vi "Engine - Copy & Script PPLTemplates.vi"(7 "CD Name":string, 8 "error in (no error)":errorcluster, 9 "RT Driver VI Path":path, 10 "RT Driver Folder Path":path, 11 "CD Source Folder Path":path) -> (0 "error out":errorcluster)   [LabVIEW 2020, in "NIVS_Consolidated_CDW_MetaDataObj.lvclass"]
doc: "Via scripting, replace the tempate RTStateVariables control with the new type def across the async and RT driver VIs, and script the compiled settings property into the constants global"
uses:
  NIVS_Consolidated_CDW_MetaDataObj.lvclass
  Common.ctl
  CD Shared lvlib.ctl
  CD Engine lvlib.ctl
  Common.vi
  CD Shared lvlib.vi
  CD Engine lvlib.vi
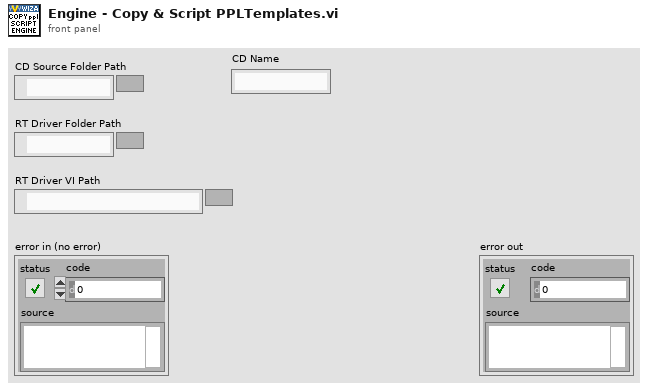
[diagram p1: front panel]
types:
  T1 = typedef "NIVS_Consolidated_CDW_MetaDataObj.lvclass/CD Engine lvlib.ctl" = enum16{"LibraryFileName", "LibraryFolderName", "Engine.FolderName", "Engine.Init.FolderName", "Engine.Run.FolderName", "Engine.Shutdown.FolderName", "Types.FolderName", "Engine.RT Driver VI.TemplatePath", "Engine.RT Driver VI.FileName", "Engine.PPL.RT Driver VI_InlineAsync.FileName", "Engine.RTStateVariables.Name", "Engine.PPL.RTStateVariables.Name", "Engine.RTStateVariables.Name.NoExtension", "Engine.Async.NameExtension", "Engine.Async.TemplateName", "Engine.PPL.Async.TemplateName", "Engine.PPL.Async.InitVSGlobals.Name", "Engine.PPL.RT Driver VI_Inline.FileName"}
  T2 = typedef "NIVS_Consolidated_CDW_MetaDataObj.lvclass/CD Shared lvlib.ctl" = enum16{"LibraryFileName", "LibraryFolderName", "ConstantsVI.VIPathAndName", "Shared.FolderName", "Shared.Types.FolderName", "Shared.Constants.VIName", "Shared.Constants.VITemplateName", "Shared.Constants.VITemplatePathAndName", "Shared.CompiledSettings.RelativePath", "Shared.Constants.RelativePath", "Shared.CompiledSettings.Name", "Shared.CompiledSettings.Name.NoExtension", "Shared.CompiledSettings.ClusterName"}
  T3 = typedef "NIVS_Consolidated_CDW_MetaDataObj.lvclass/Common.ctl" = enum16{"ProjectName", "TemplatesFolderName", "PPLTemplatesFolderName", "ProjectTemplatePathAndName", "ProjectPPLTemplatePathAndName", "TimingAndSyncFolderName", "CustomDeviceFolderName", "PathToTemplates", "PathToPPLTemplates", "PathToExplorerPPLTemplates", "PathToEnginePPLTemplates", "PathToConfigurationFile", "ProjectConfigurationName"}
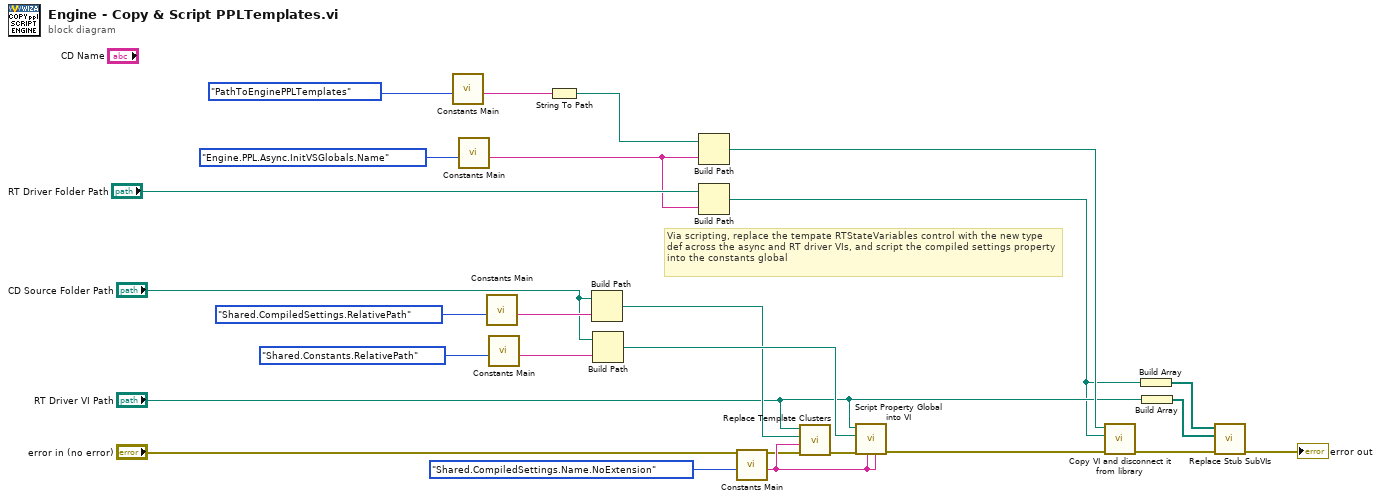
[diagram p0: block diagram]
diagram:
  # "Via scripting, replace the tempate RTStateVariables control with the new type def across the async and RT driver VIs, and script the compiled settings property into the constants global"
  n1 = call-poly "Constants Main.vi"("Action"=Common."PathToEnginePPLTemplates") -> ("Output"=w22:string)  [unwired: 10 in]
  n2 = call-poly "Constants Main.vi"("Action"=CD_Engine_lvlib."Engine.PPL.Async.InitVSGlobals.Name") -> ("Output"=w8:string)  [unwired: 10 in]
  n3 = call-poly "Constants Main.vi"("Action"=CD_Shared_lvlib."Shared.CompiledSettings.RelativePath") -> ("Output"=w19:string)  [unwired: 10 in]
  n4 = call-poly "Constants Main.vi"("Action"=CD_Shared_lvlib."Shared.Constants.RelativePath") -> ("Output"=w17:string)  [unwired: 10 in]
  n5 = String To Path(string=w22) -> (path=w11:path)
  n6 = Build Path(base path="CD Source Folder Path", name or relative path=w19) -> (appended path=w24:path)
  n7 = Build Path(base path="CD Source Folder Path", name or relative path=w17) -> (appended path=w25:path)
  n8 = Build Path(base path=w11, name or relative path=w8) -> (appended path=w10:path)
  n9 = Build Path(base path="RT Driver Folder Path", name or relative path=w8) -> (appended path=w2:path)
  n10 = call-poly "Constants Main.vi"("Action"=CD_Shared_lvlib."Shared.CompiledSettings.Name.NoExtension") -> ("Output"=w14:string)  [unwired: 10 in]
  n11 = call "Replace Template Clusters.vi"("error in (no error)"="error in (no error)", "Control Name"=w14, "Path to Cluster to Replace"=w24, "Path to VI"="RT Driver VI Path") -> ("error out"=w23:errorcluster)  [unwired: 7 in]
  n12 = call "Script Property Global into VI.vi"("GlobalControlName"=w14, "StringConstantToReplace"=w14, "error in (no error)"=w23, "Path to Global"=w25, "Path to VI"="RT Driver VI Path") -> ("error out"=w1:errorcluster)  [unwired: 6 in]
  n13 = call "Copy VI and disconnect it from library.vi"("error in (no error)"=w1, "VI Target Path"=w2, "VI Source Path"=w10) -> ("error out"=w7:errorcluster)  [unwired: 8 in]
  n14 = Build Array(w2) -> (w3:path[])
  n15 = Build Array("RT Driver VI Path") -> (w4:path[])
  n16 = call "Replace Stub SubVIs.vi"("error in"=w7, "VIs to Process"=w4, "subVIs to replace"=w3) -> ("error out"=→"error out":errorcluster)  [unwired: 8 in]
